vi "Get Ports.vi"() -> (0 "Array":string[](array[string]), 3 "find list":string[](array[string]))   [LabVIEW 2019]
doc: "Finds all devices connected to the PC through GPIB, USBTMC, or RS232 (COM ports).\nReturns as list of the connected devices' model numbers as well as their addresses"
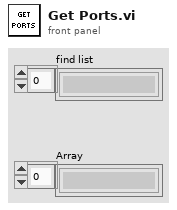
[diagram p1: front panel]
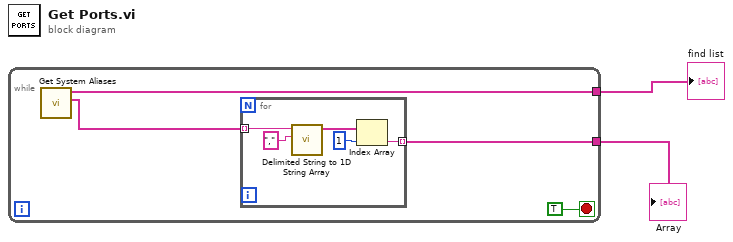
[diagram p0: block diagram]
diagram:
  n1 = while {
    tunnel: [w4] -> w1
    tunnel: [w6] -> w2
    stop <- TRUE stop-if-true
    n2 = call <userlib>:"Get System Aliases.vi"() -> ("Equipment Response"=w5:string[], "find list"=w6:string[])  [unwired: 9 in, 1 out]
    n3 = for {
      tunnel: w5 -> [w11] mode=indexing
      tunnel: [w7] -> w4 mode=indexing
      n4 = call <vilib>:"Delimited String to 1D String Array.vi"("delimiter"=",", "delimited string"=w11) -> ("string array"=w9:string[])  [unwired: 9 in]
      n5 = Index Array(array=w9, index=1) -> (element=w7:string)
    }
  }
  "find list" <- w2
  "Array" <- w1
